vi "LED_no_wait.vi"(1 "Testpulser On/Off":bool, 3 "Testpulse Separation (20 ns ticks)":u32=500, 4 "Testpulse duration (20 ns ticks)":u32=1) -> (0 "Is Test Pulse?":bool)   [LabVIEW 2012]
uses:
  <vilib>/rvi/eio/common/nirviEmuTemplateMethod_errors.vi
  <vilib>/eio/EIONode/EIONode.xnode
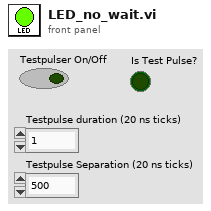
[diagram p1: front panel]
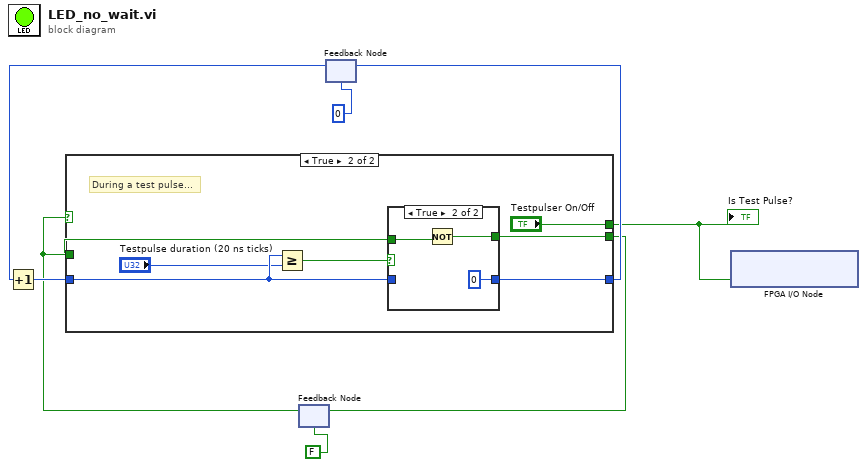
[diagram p0: block diagram]
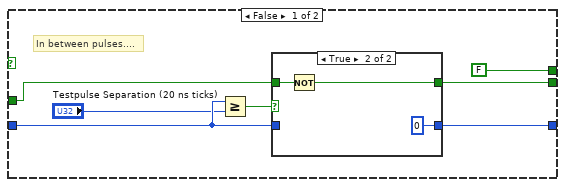
[diagram p2: hidden frame]
diagram:
  n1 = feedback #1(FALSE) -> (w3:bool)
  n2 = feedback #2(u32 0) -> (w6:u32)
  n3 = Increment(x=w6) -> (x+1=w8:u32)
  n4 = case shown="True" w3 {
    tunnel: w8 -> [w12 w24]
    tunnel: [w15 w26] -> w5
    tunnel: [w14 w27] -> w2
    tunnel: [FALSE ("IO Module\\D0 0") "Testpulser On/Off"] -> w1
    tunnel: w3 -> [w9 w21]
    frame False {
      # "In between pulses...."
      n5 = Greater Or Equal?(x=w12, y="Testpulse Separation (20 ns ticks)") -> (x >= y?=w11:bool)
      n6 = case shown="True" w11 {
        tunnel: [w17 u32 0] -> w15
        tunnel: w12 -> [w17 _]
        tunnel: [w16 w19] -> w14
        tunnel: w9 -> [w16 w18]
        frame False {
        }
        frame True {
          n7 = Not(x=w18) -> (.not. x?=w19:bool)
        }
      }
    }
    frame True {
      # "During a test pulse..."
      n8 = Greater Or Equal?(x=w24, y="Testpulse duration (20 ns ticks)") -> (x >= y?=w23:bool)
      n9 = case shown="True" w23 {
        tunnel: w24 -> [w29 _]
        tunnel: [w28 w32] -> w27
        tunnel: [w29 u32 0] -> w26
        tunnel: w21 -> [w28 w30]
        frame False {
        }
        frame True {
          n10 = Not(x=w30) -> (.not. x?=w32:bool)
        }
      }
    }
  }
  "Is Test Pulse?" <- w1
  n11 = feedback-in #1(w2) -> ()
  n12 = feedback-in #2(w5) -> ()
  n13 = xnode "FPGA I/O Node"("IO Module\\D0 0"=w1) -> ()  [unwired: 1 in, 1 out]
